vi "Get_Sample_ID.vi"(8 "error in (no error)":errorcluster, 11 "DB in":refnum<class "DB.lvclass">) -> (0 "error out":errorcluster, 1 "Sample_ID":string="0", 2 "Sample_ID":i16, 3 "DB out":refnum<class "DB.lvclass">)   [LabVIEW 2019, in "DB.lvclass"]
uses:
  DB.lvclass
  DB.lvclass/DB.ctl
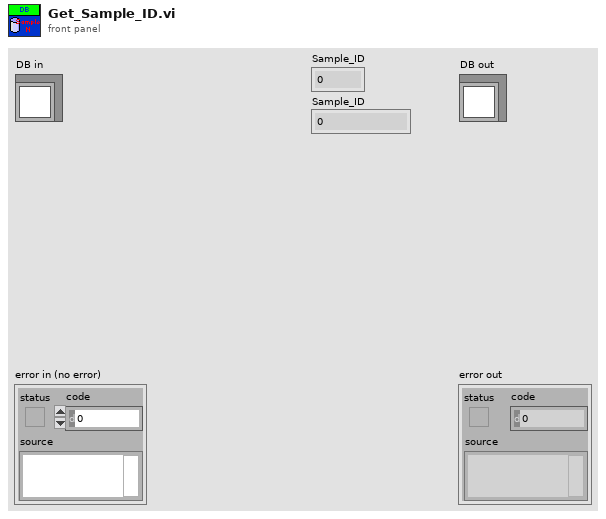
[diagram p1: front panel]
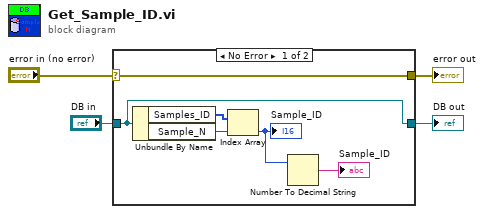
[diagram p0: block diagram]
diagram:
  n1 = case shown="No Error" "error in (no error)" {
    selector: "error in (no error)" -> [w10 w12]
    tunnel: [w10 w12] -> w3
    tunnel: [w9 w11] -> w1
    tunnel: "DB in" -> [w9 w11]
    frame No Error {
      n2 = Unbundle By Name(w9) -> ("Samples_ID"=w8:i16[], "Sample_N"=w7:i16)
      n3 = Index Array(array=w8, index=w7) -> (element=w6:i16)
      "Sample_ID" <- w6
      n4 = Number To Decimal String(number=w6) -> (decimal integer string=→"Sample_ID":string)  [unwired: 1 in]
    }
    frame Error {
    }
  }
  "error out" <- w3
  "DB out" <- w1
